vi "Read Handle Activate Menu Msg.vi"(11 "File Explorer Event Filter in":refnum<class "File Explorer Event Filter.lvclass">) -> (3 "File Explorer Event Filter out":refnum<class "File Explorer Event Filter.lvclass">, 4 "Handle Activate Menu On Tree Item Msg":refnum<class "Handle Activate Menu On Tree Item Msg.lvclass">)   [LabVIEW 2017, in "File Explorer.lvlib" / "File Explorer Event Filter.lvclass"]
uses:
  <vilib>/gpm_packages/@cs/file-explorer-extension/Source/File Explorer/File Explorer Event Filter/File Explorer Event Filter.lvclass
  <vilib>/gpm_packages/@cs/file-explorer-extension/Source/File Explorer/File Explorer Messages/Handle Activate Menu On Tree Item Msg/Handle Activate Menu On Tree Item Msg.lvclass
  <vilib>/gpm_packages/@cs/file-explorer-extension/Source/File Explorer/File Explorer Event Filter/File Explorer Event Filter.lvclass/File Explorer Event Filter.ctl
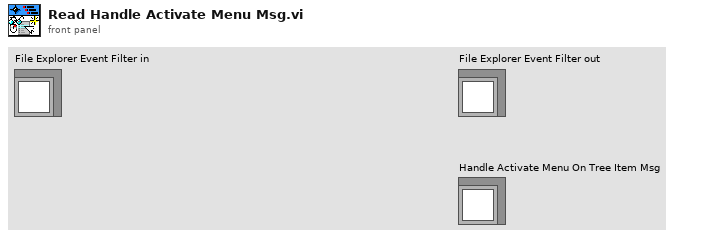
[diagram p1: front panel]
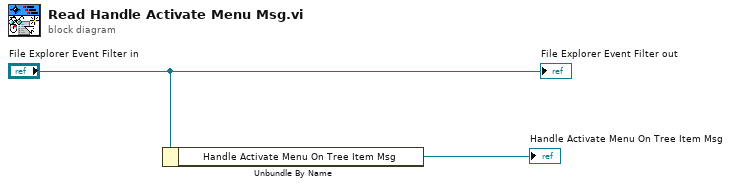
[diagram p0: block diagram]
diagram:
  n1 = Unbundle By Name("File Explorer Event Filter in") -> ("Handle Activate Menu On Tree Item Msg"=→"Handle Activate Menu On Tree Item Msg":refnum<class "Handle Activate Menu On Tree Item Msg.lvclass">)
  "File Explorer Event Filter out" <- "File Explorer Event Filter in"
